vi "Fetch Cal Standards.vi"(0 "ACM4509 in":refnum<class "Cal Standard.lvclass">, 11 "error in (no error)":errorcluster) -> (4 "ACM4509 out":refnum<class "Cal Standard.lvclass">, 15 "error out":errorcluster)   [LabVIEW 2023, in "ACM 4509 Cal Standard.lvlib" / "Cal Standard.lvclass"]
uses:
  Cal Standard.lvclass
  C:/srd-semi-rfcal-software/AuxTools/STSRFFixtureCharactUtility/Source/Code Modules/Fixture/Instruments/Cal Standard/Cal Standard Base/Cal Standard Base.lvclass
  Cal Standard.lvclass/Cal Standard.ctl
  Dependencies/ACM/API/Controls/ACM S-Parameters.ctl
  Instruments/Cal Standard/Type Definitions/One-Port Cal Standard.ctl
  Instruments/Cal Standard/Type Definitions/One-Port Charact Data.ctl
  Instruments/Cal Standard/Type Definitions/Standard Type.ctl
  Properties/Read Resource Name.vi
  Instruments/Cal Standard/Cal Standard Base/Properties/Write One-Port Cal Standards.vi
  Dependencies/ACM/ACM Visa Driver.lvlib
  Instruments/RFFixtureCharact.Instruments.lvlib
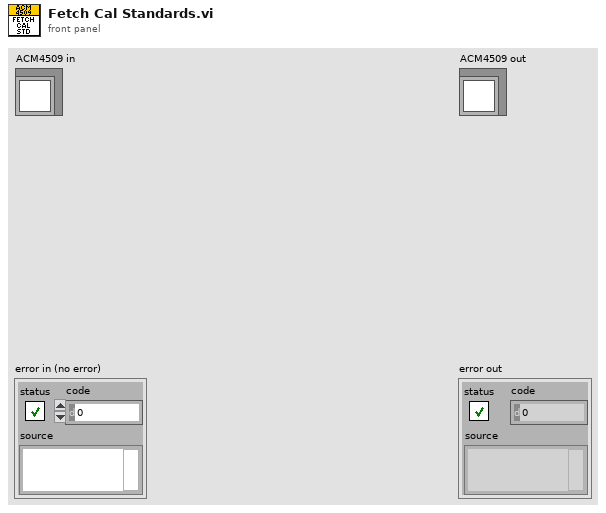
[diagram p1: front panel]
types:
  T1 = typedef "RFFixtureCharact.Instruments.lvlib/One-Port Cal Standard.ctl" = cluster{"Port Name":string, "Charact Data":T2[]}
  T2 = typedef "RFFixtureCharact.Instruments.lvlib/One-Port Charact Data.ctl" = cluster{"Standard Type":T3, "Frequencies":dbl[], "S11":cdb[]}
  T3 = typedef "RFFixtureCharact.Instruments.lvlib/Standard Type.ctl" = enum16{"Short", "Open", "Load"}
  T4 = typedef "ACM Visa Driver.lvlib/ACM S-Parameters.ctl" = string
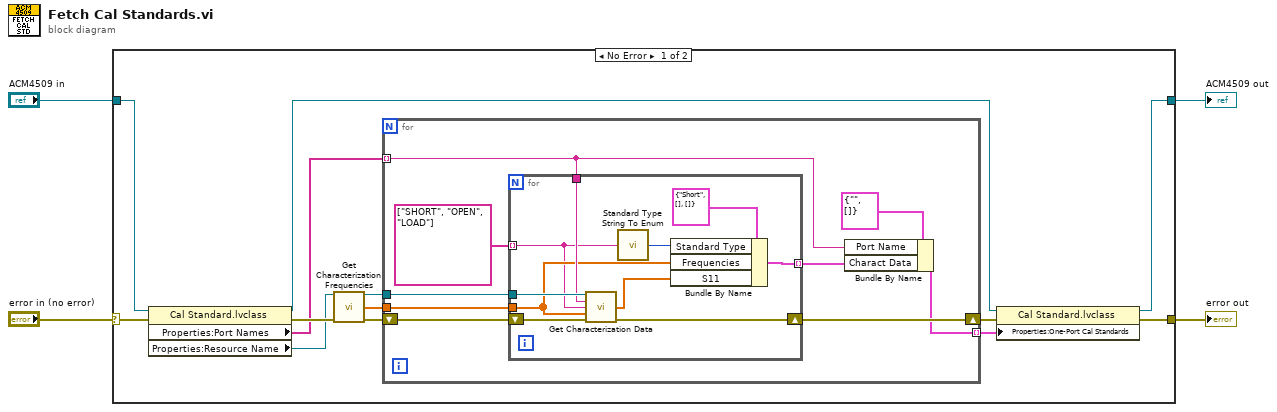
[diagram p0: block diagram]
diagram:
  n1 = case shown="No Error" "error in (no error)" {
    selector: "error in (no error)" -> [w10 w38]
    tunnel: [w13 w38] -> w3
    tunnel: [w12 w37] -> w1
    tunnel: "ACM4509 in" -> [w8 w37]
    frame No Error {
      n2 = property class="Cal Standard.lvclass"(reference=w8, error in=w10) -> (reference out=w7:refnum<class "Cal Standard.lvclass">, error out=w9:errorcluster, "Properties:Port Names"=w6:string[], "Properties:Resource Name"=w5:refnum<visa-resource-name>)
      n3 = call "Get Characterization Frequencies.vi"("VISA resource name"=w5, "error in (no error)"=w9) -> ("VISA resource name out"=w17:refnum<visa-resource-name>, "S-Par Characterization Frequencies"=w16:dbl[], "error out"=w15:errorcluster)  [unwired: 11 in]
      n4 = for {
        tunnel: w17 -> [w26]
        tunnel: w16 -> [w25]
        shift-right: [w23] -> w14
        shift-left: w15 -> [w24]
        tunnel: w6 -> [w19] mode=indexing
        tunnel: [w18] -> w11 mode=indexing
        n5 = for {
          tunnel: w26 -> [w36]
          tunnel: w25 -> [w32]
          shift-right: [w30] -> w23
          shift-left: w24 -> [w35]
          tunnel: w19 -> [w34]
          tunnel: T4[] ["SHORT", "OPEN", "LOAD"] -> [w29] mode=indexing
          tunnel: [w27] -> w20 mode=indexing
          n6 = call "Get Characterization Data.vi"("VISA resource name"=w36, "ACM Path"=w34, "S-Parameter"=w29, "Characterization Frequencies (for Temp Co)"=w32, "error in (no error)"=w35) -> ("S-Par Characterization Data"=w31:cdb[], "error out"=w30:errorcluster)  [unwired: 8 in, 1 out]
          n7 = call "Standard Type String To Enum.vi"("Standard Type"=w29) -> ("Standard Type"=w28:T3)
          n8 = Bundle By Name(cluster=T2 {"Standard Type"=enum."Short", "Frequencies"=[], "S11"=[]} ("Cal Characterization Data"), "Standard Type"=w28, "Frequencies"=w32, "S11"=w31) -> (w27:T2)
        }
        n9 = Bundle By Name(cluster=T1 {"Port Name"="", "Charact Data"=[]} ("One-Port Cal Standard"), "Port Name"=w19, "Charact Data"=w20) -> (w18:T1)
      }
      n10 = property class="Cal Standard.lvclass"(reference=w7, error in=w14, "Properties:One-Port Cal Standards"=w11) -> (reference out=w12:refnum<class "Cal Standard.lvclass">, error out=w13:errorcluster)
    }
    frame Error {
    }
  }
  "error out" <- w3
  "ACM4509 out" <- w1
